vi "TestExec.Config, Get Station VI Path.vi"() -> (0 "error out":errorcluster, 2 "Child VI Name":string, 3 "Sta VI Path":path)   [LabVIEW 2018]
uses:
  <vilib>/Utility/config.llb/Read Key (String).vi
  <vilib>/Utility/config.llb/NI_LVConfig.lvlib
  <vilib>/KATE/Files/File Utils.lvlib
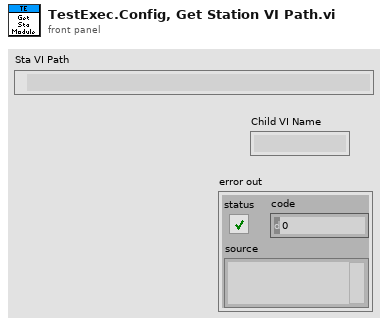
[diagram p1: front panel]
types:
  T1 = enum32{"invalid app kind", "Development System", "Run Time System", "Student Edition", "Embedded LabVIEW", "Evaluation", "Custom"}
  T2 = typedef "NI_LVConfig.lvlib/Config Data RefNum.ctl" = refnum<k1>
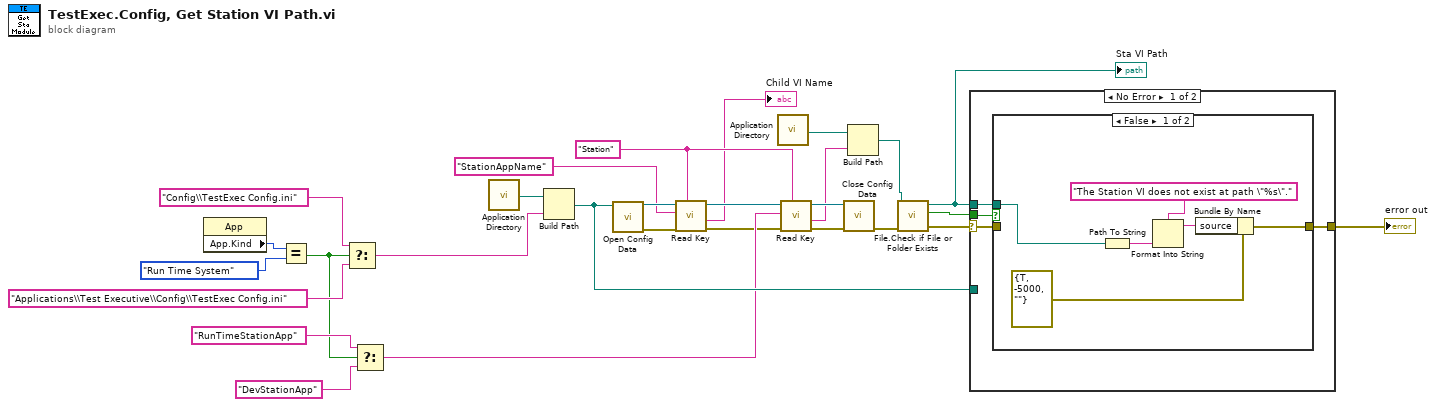
[diagram p0: block diagram]
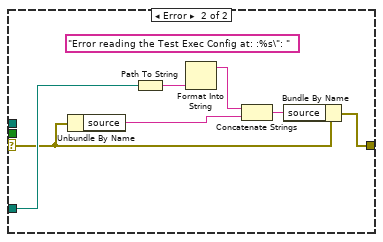
[diagram p3: hidden frame]
diagram:
  w10 = "Station" ("section")
  n1 = property class="App"() -> ("App.Kind"=w7:T1)  [unwired: 2 in, 2 out]
  n2 = Equal?(x=w7, y=T1."Run Time System" ("Application:Kind")) -> (x = y?=w2:bool)
  n3 = Select(t="Config\\TestExec Config.ini", s=w2, f="Applications\\Test Executive\\Config\\TestExec Config.ini") -> (s? t:f=w3:string)
  n4 = Select(t="RunTimeStationApp" ("key"), s=w2, f="DevStationApp" ("key")) -> (s? t:f=w15:string)
  n5 = call <vilib>:"Application Directory.vi"() -> ("Application Directory"=w1:path)
  n6 = Build Path(base path=w1, name or relative path=w3) -> (appended path=w21:path)
  n7 = call <vilib>:"Open Config Data.vi"("configuration file path"=w21) -> ("error out"=w13:errorcluster, "refnum"=w14:T2)  [unwired: 8 in, 1 out]
  n8 = call-poly <vilib>:"Read Key.vi"("section"=w10, "error in (no error)"=w13, "key"="StationAppName" ("section"), "refnum"=w14) -> ("error out"=w12:errorcluster, "value"=→"Child VI Name":string, "refnum out"=w11:T2)  [unwired: 4 in, 1 out]
  n9 = call <vilib>:"Application Directory.vi"() -> ("Application Directory"=w20:path)
  n10 = call-poly <vilib>:"Read Key.vi"("section"=w10, "error in (no error)"=w12, "key"=w15, "refnum"=w11) -> ("error out"=w27:errorcluster, "value"=w18:string, "refnum out"=w28:T2)  [unwired: 4 in, 1 out]
  n11 = call <vilib>:"Close Config Data.vi"("error in (no error)"=w27, "refnum"=w28) -> ("error out"=w26:errorcluster)  [unwired: 8 in, 1 out]
  n12 = Build Path(base path=w20, name or relative path=w18) -> (appended path=w19:path)
  n13 = call <vilib>:"File.Check if File or Folder Exists.vi"("error in"=w26, "Path"=w19) -> ("error out"=w25:errorcluster, "Exists"=w24:bool, "Dup Path"=w22:path)  [unwired: 5 in, 2 out]
  "Sta VI Path" <- w22
  n14 = case shown="No Error" w25 {
    selector: w25 -> [w30 w41]
    tunnel: w24 -> [w32 _]
    tunnel: w22 -> [w31 _]
    tunnel: [w29 w40] -> w23
    tunnel: w21 -> [_ w45]
    frame No Error {
      n15 = case shown="False" w32 {
        tunnel: w31 -> [w34 _]
        tunnel: w30 -> [_ w39]
        tunnel: [w33 w39] -> w29
        frame False {
          n16 = Path To String(path=w34) -> (string=w38:string)
          n17 = Format Into String(format string="The Station VI does not exist at path \"%s\".", w38) -> (resulting string=w36:string)  [unwired: 2 in, 1 out]
          n18 = Bundle By Name(cluster=errorcluster {"status"=TRUE, "code"=-5000, "source"=""} ("error constant"), "source"=w36) -> (w33:errorcluster)
        }
        frame True {
        }
      }
    }
    frame Error {
      (unwired) "Error reading the Test Exec Config at: :%s\": "
      n19 = Unbundle By Name(w41) -> ("source"=w43:string)
      n20 = Path To String(path=w45) -> (string=w46:string)
      n21 = Format Into String(w46) -> (resulting string=w44:string)  [unwired: 3 in, 1 out]
      n22 = Concatenate Strings(w44, w43) -> (w42:string)
      n23 = Bundle By Name(cluster=w41, "source"=w42) -> (w40:errorcluster)
    }
  }
  "error out" <- w23
